vi "Send String.vi"(8 "error in (no error)":errorcluster, 9 "MAMP2":u32, 10 "RES":u8=1, 11 "RAMP":u8=1) -> (0 "error out":errorcluster, 3 "Message":string)   [LabVIEW 2017]
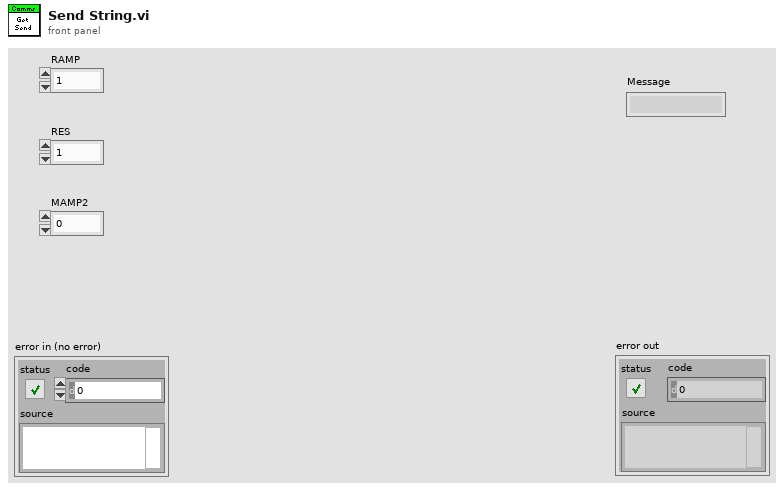
[diagram p1: front panel]
types:
  T1 = enum16{"Init", "Get Index", "Analyze Part", "Analyze Prts", "Analyze Prta", "Set VER", "Set TYPE"}
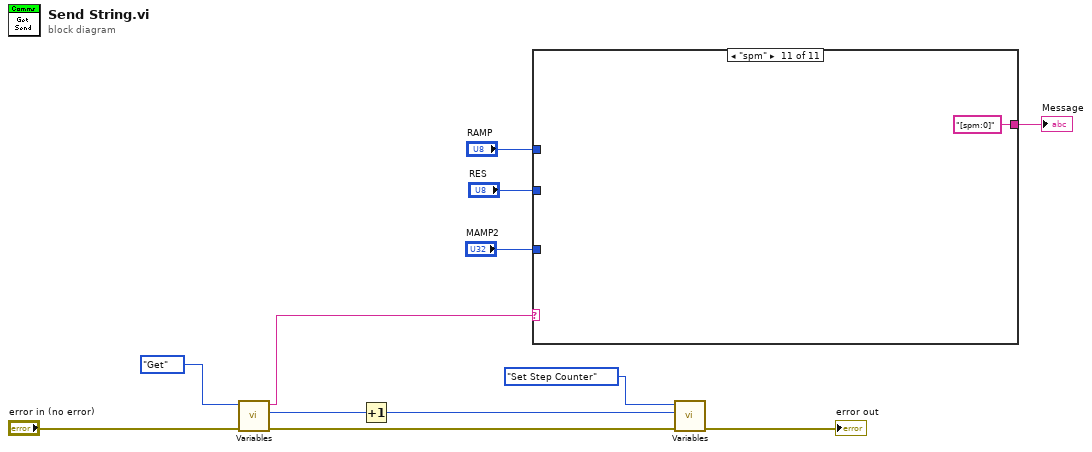
[diagram p0: block diagram]
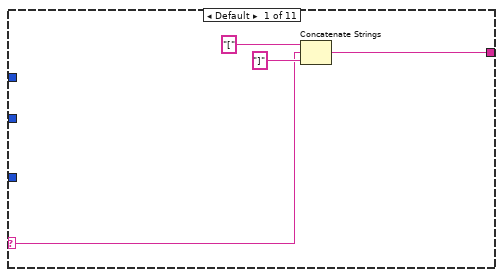
[diagram p2: hidden frame]
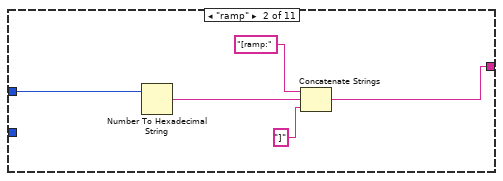
[diagram p3: hidden frame]
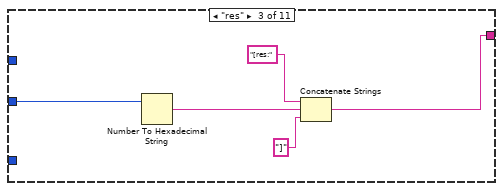
[diagram p4: hidden frame]
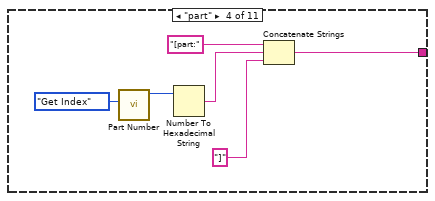
[diagram p5: hidden frame]
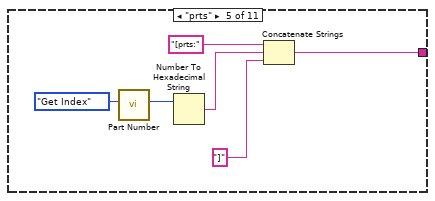
[diagram p6: hidden frame]
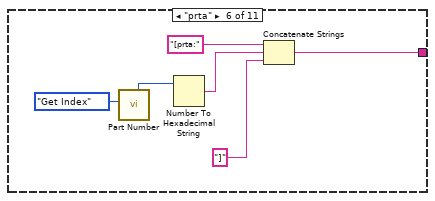
[diagram p7: hidden frame]
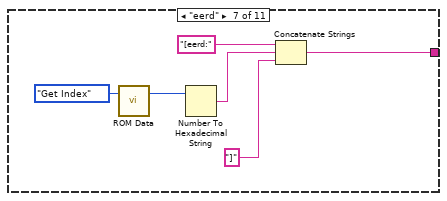
[diagram p8: hidden frame]
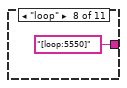
[diagram p9: hidden frame]
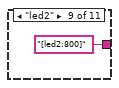
[diagram p10: hidden frame]
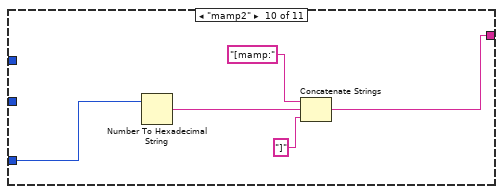
[diagram p11: hidden frame]
diagram:
  n1 = call "Variables.vi"("error in (no error)"="error in (no error)", "Command"=enum16{"Init", "Get", "Set Step Counter"}."Get") -> ("error out"=w9:errorcluster, "Step Counter"=w4:i32, "Out Message"=w2:string)  [unwired: 7 in]
  n2 = Increment(x=w4) -> (x+1=w3:i32)
  n3 = case shown="\"spm\"" w2 {
    selector: w2 -> [w14 _ _ _ _ _ _ _ _ _ _]
    tunnel: [w13 w18 w24 w29 w35 w41 w47 "[loop:5550]" "[led2:800]" w55 "[spm:0]"] -> w10
    tunnel: "RES" -> [_ _ w22 _ _ _ _ _ _ _ _]
    tunnel: "RAMP" -> [_ w21 _ _ _ _ _ _ _ _ _]
    tunnel: "MAMP2" -> [_ _ _ _ _ _ _ _ _ w53 _]
    frame Default {
      n4 = Concatenate Strings("[" ("string"), w14, "]" ("string")) -> (w13:string)
    }
    frame "ramp" {
      n5 = Number To Hexadecimal String(2:w21) -> (0:w20:string)  [unwired: 1 in]
      n6 = Concatenate Strings("[ramp:", w20, "]" ("string")) -> (w18:string)
    }
    frame "res" {
      n7 = Number To Hexadecimal String(2:w22) -> (0:w26:string)  [unwired: 1 in]
      n8 = Concatenate Strings("[res:", w26, "]" ("string")) -> (w24:string)
    }
    frame "part" {
      n9 = call "Part Number.vi"("Command"=T1."Get Index") -> ("Part Index"=w28:i32)  [unwired: 5 in, 5 out]
      n10 = Number To Hexadecimal String(2:w28) -> (0:w31:string)  [unwired: 1 in]
      n11 = Concatenate Strings("[part:", w31, "]" ("string")) -> (w29:string)
    }
    frame "prts" {
      n12 = call "Part Number.vi"("Command"=T1."Get Index") -> ("Prts Index"=w34:i32)  [unwired: 5 in, 5 out]
      n13 = Number To Hexadecimal String(2:w34) -> (0:w37:string)  [unwired: 1 in]
      n14 = Concatenate Strings("[prts:", w37, "]" ("string")) -> (w35:string)
    }
    frame "prta" {
      n15 = call "Part Number.vi"("Command"=T1."Get Index") -> ("Prta Index"=w39:i32)  [unwired: 5 in, 5 out]
      n16 = Number To Hexadecimal String(2:w39) -> (0:w43:string)  [unwired: 1 in]
      n17 = Concatenate Strings("[prta:", w43, "]" ("string")) -> (w41:string)
    }
    frame "eerd" {
      n18 = call "ROM Data.vi"("Command"=enum16{"Init", "Get Index", "Analyze"}."Get Index") -> ("Index"=w46:i32)  [unwired: 1 in, 1 out]
      n19 = Number To Hexadecimal String(2:w46) -> (0:w49:string)  [unwired: 1 in]
      n20 = Concatenate Strings("[eerd:", w49, "]" ("string")) -> (w47:string)
    }
    frame "loop" {
    }
    frame "led2" {
    }
    frame "mamp2" {
      n21 = Number To Hexadecimal String(2:w53) -> (0:w57:string)  [unwired: 1 in]
      n22 = Concatenate Strings("[mamp:", w57, "]" ("string")) -> (w55:string)
    }
    frame "spm" {
    }
  }
  "Message" <- w10
  n23 = call "Variables.vi"("error in (no error)"=w9, "Value"=w3, "Command"=enum16{"Init", "Get", "Set Step Counter"}."Set Step Counter") -> ("error out"=→"error out":errorcluster)  [unwired: 6 in, 2 out]
